vi "SaveFFTDataSet.vi"(6 "AssetNodeMap":variant, 7 "do not write to database":bool, 8 "error in (no error)":errorcluster, 9 "MCSA FFT":T1, 10 "DataSetRegistry":T2, 11 "event in":T4) -> (0 "error out":errorcluster, 3 "event out":T4)   [LabVIEW 2017, in "McsaDataEventCreator.lvlib"]
uses:
  <vilib>/addons/InsightCM/Devices/Shared/Mcsa/McsaDataEventCreator/McsaDataEventCreator.lvlib
  <vilib>/addons/InsightCM/Devices/Shared/Common/DataEvent/controls/Event.ctl
  <vilib>/addons/InsightCM/MessageBus/Base/controls/DataEvent.ctl
  <vilib>/addons/InsightCM/MessageBus/Base/controls/KeyValuePair.ctl
  <vilib>/addons/InsightCM/Devices/Shared/Common/DataEvent/controls/DataSet.ctl
  <vilib>/addons/InsightCM/MessageBus/Base/controls/DataSetMetadata.ctl
  <vilib>/addons/InsightCM/MessageBus/Base/controls/TrendPoint.ctl
  <vilib>/addons/InsightCM/MessageBus/Base/controls/TrendAlarmUpdate.ctl
  <vilib>/addons/InsightCM/MessageBus/Base/controls/TrendAlarmTransition.ctl
  <vilib>/addons/InsightCM/Devices/Shared/Mcsa/McsaDataEventCreator/controls/Registry_DataSet.ctl
  <vilib>/addons/InsightCM/Devices/Shared/Mcsa/McsaDataEventCreator/controls/DataSetType.ctl
  <vilib>/addons/InsightCM/Utilities/Analysis/MCSA/controls/McsaFFT.ctl
  <vilib>/addons/InsightCM/Devices/Shared/Common/DataEvent/DataEvent.lvlib
  <vilib>/addons/InsightCM/Utilities/Analysis/MCSA/McsaAnalysisFunctions.lvlib
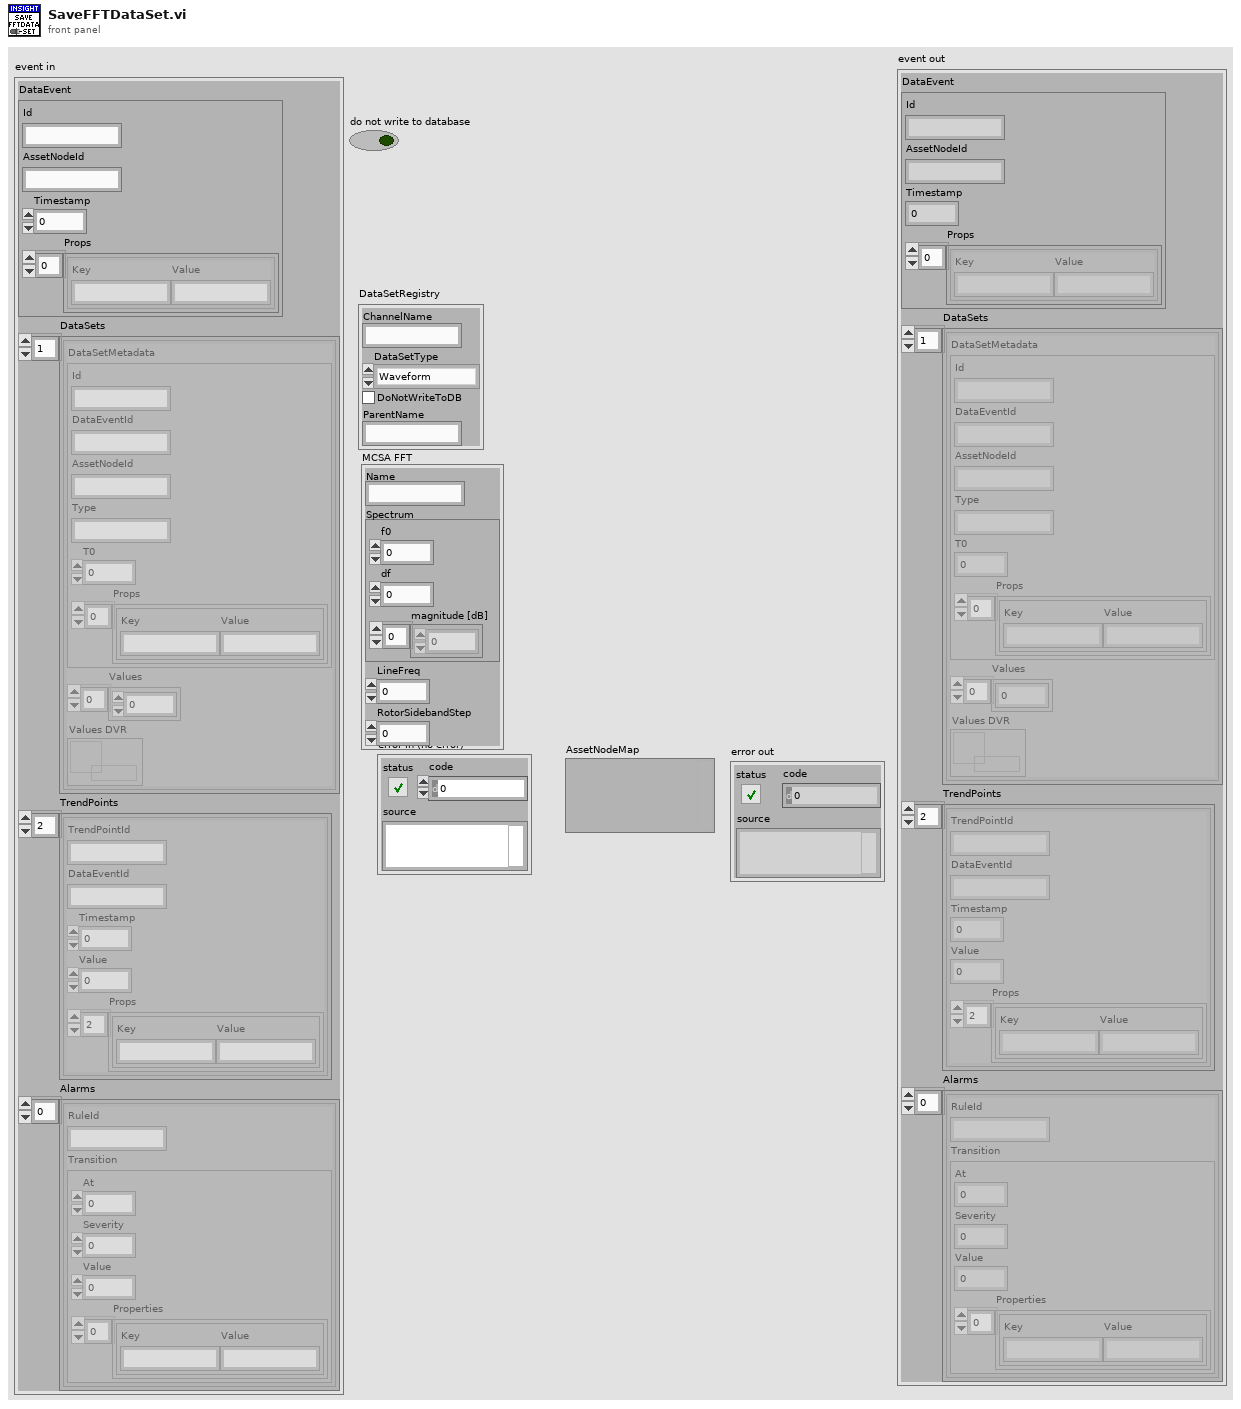
[diagram p1: front panel]
types:
  T1 = typedef "McsaAnalysisFunctions.lvlib/McsaFFT.ctl" = cluster{"Name":string, "Spectrum":cluster{"f0":dbl, "df":dbl, "magnitude [dB]":dbl[]}, "LineFreq":dbl, "RotorSidebandStep":dbl}
  T2 = typedef "McsaDataEventCreator.lvlib/Registry_DataSet.ctl" = cluster{"ChannelName":string, "DataSetType":T3, "DoNotWriteToDB":bool, "ParentName":string}
  T3 = typedef "McsaDataEventCreator.lvlib/DataSetType.ctl" = enum16{"Waveform", "MCSAFFT", "TorqueWFM"}
  T4 = typedef "DataEvent.lvlib/Event.ctl" = cluster{"DataEvent":T5, "DataSets":T7[], "TrendPoints":T9[], "Alarms":T10[]}
  T5 = typedef "DataEvent.ctl" = cluster{"Id":string, "AssetNodeId":string, "Timestamp":i64, "Props":T6[]}
  T6 = typedef "KeyValuePair.ctl" = cluster{"Key":string, "Value":string}
  T7 = typedef "DataEvent.lvlib/DataSet.ctl" = cluster{"DataSetMetadata":T8, "Values":sgl[], "Values DVR":refnum<data-value>}
  T8 = typedef "DataSetMetadata.ctl" = cluster{"Id":string, "DataEventId":string, "AssetNodeId":string, "Type":string, "T0":i64, "Props":T6[]}
  T9 = typedef "TrendPoint.ctl" = cluster{"TrendPointId":string, "DataEventId":string, "Timestamp":i64, "Value":dbl, "Props":T6[]}
  T10 = typedef "TrendAlarmUpdate.ctl" = cluster{"RuleId":string, "Transition":T11}
  T11 = typedef "TrendAlarmTransition.ctl" = cluster{"At":i64, "Severity":i32, "Value":dbl, "Properties":T6[]}
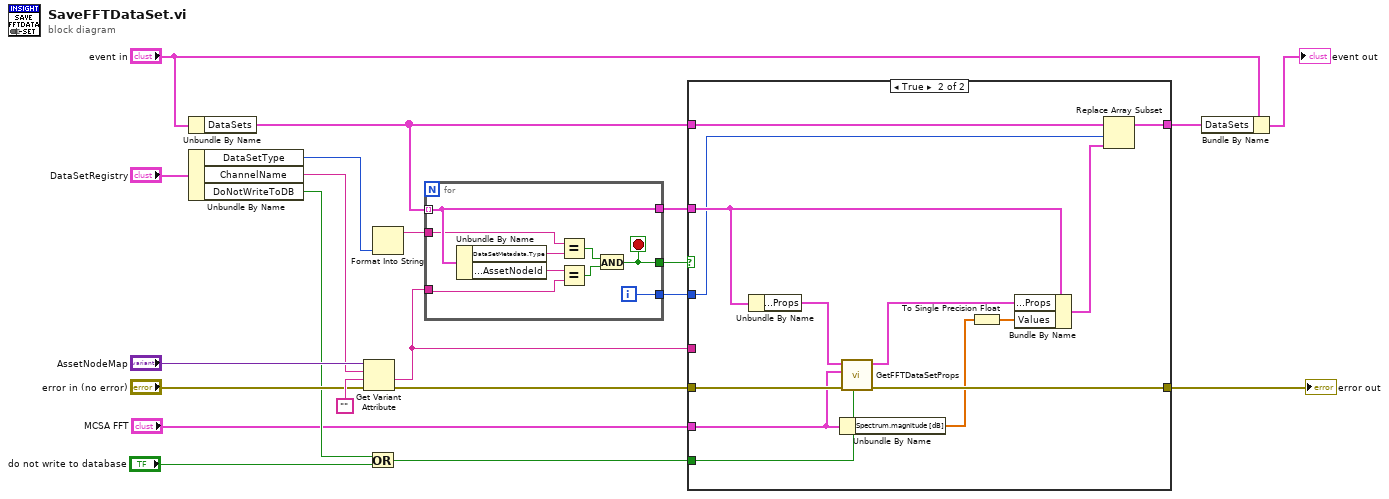
[diagram p0: block diagram]
diagram:
  n1 = Unbundle By Name("event in") -> ("DataSets"=w15:T7[])
  n2 = Unbundle By Name("DataSetRegistry") -> ("DataSetType"=w8:T3, "ChannelName"=w1:string, "DoNotWriteToDB"=w5:bool)
  n3 = Get Variant Attribute(Variant="AssetNodeMap", name=w1, default value (empty Variant)="", error in="error in (no error)") -> (value=w17:string, error out=w7:errorcluster)  [unwired: 2 out]
  n4 = Or(x=w5, y="do not write to database") -> (x .or. y?=w4:bool)
  n5 = Format Into String(w8) -> (resulting string=w2:string)  [unwired: 3 in, 1 out]
  n6 = for {
    tunnel: w15 -> [w28] mode=indexing
    tunnel: w17 -> [w29]
    tunnel: [w24] -> w18
    tunnel: [w28] -> w12
    tunnel: [w27] -> w11
    tunnel: w2 -> [w22]
    i -> [w27]
    stop <- w24 stop-if-true
    n7 = Unbundle By Name(w28) -> ("DataSetMetadata.Type"=w23:string, "DataSetMetadata.AssetNodeId"=w30:string)
    n8 = Equal?(x=w22, y=w23) -> (x = y?=w26:bool)
    n9 = Equal?(x=w30, y=w29) -> (x = y?=w25:bool)
    n10 = And(x=w26, y=w25) -> (x .and. y?=w24:bool)
  }
  n11 = case shown="True" w18 {
    tunnel: w7 -> [w31 w40]
    tunnel: w17 -> [_ _]
    tunnel: w15 -> [w32 w44]
    tunnel: [w32 w43] -> w14
    tunnel: w12 -> [_ w45]
    tunnel: w11 -> [_ w42]
    tunnel: [w31 w39] -> w9
    tunnel: "MCSA FFT" -> [_ w35]
    tunnel: w4 -> [_ w36]
    frame False {
    }
    frame True {
      n12 = Unbundle By Name(w45) -> ("DataSetMetadata.Props"=w37:T6[])
      n13 = Unbundle By Name(w35) -> ("Spectrum.magnitude [dB]"=w34:dbl[])
      n14 = call <vilib>:"GetFFTDataSetProps.vi"("do not write to database"=w36, "error in (no error)"=w40, "MCSA FFT"=w35, "dataset props in"=w37) -> ("error out"=w39:errorcluster, "dataset props out"=w38:T6[])  [unwired: 6 in]
      n15 = To Single Precision Float(number=w34) -> (single precision float=w33:sgl[])
      n16 = Bundle By Name(cluster=w45, "DataSetMetadata.Props"=w38, "Values"=w33) -> (w41:T7)
      n17 = Replace Array Subset(array=w44, new element=w41, index=w42) -> (w43:T7[])
    }
  }
  "error out" <- w9
  n18 = Bundle By Name(cluster="event in", "DataSets"=w14) -> (→"event out":T4)
